vi "motor_stepping_diag_correct.vi"(0 "Initial Voltage (V)":dbl, 1 "Voltage Step (V)":dbl, 2 "First?":bool, 3 "Steps":dbl, 5 "Final Voltage (V)":dbl, 7 "Actual Voltage (V)  in":dbl, 9 "Final Voltage (V) 2":dbl, 11 "error in (no error)":errorcluster, 12 "Voltage Step2":dbl, 14 "Physical Channel":tag="Dev1/ao0") -> (4 "Actual Voltage (V)":dbl, 6 "Boolean":bool, 15 "error out":errorcluster)   [LabVIEW 2015]
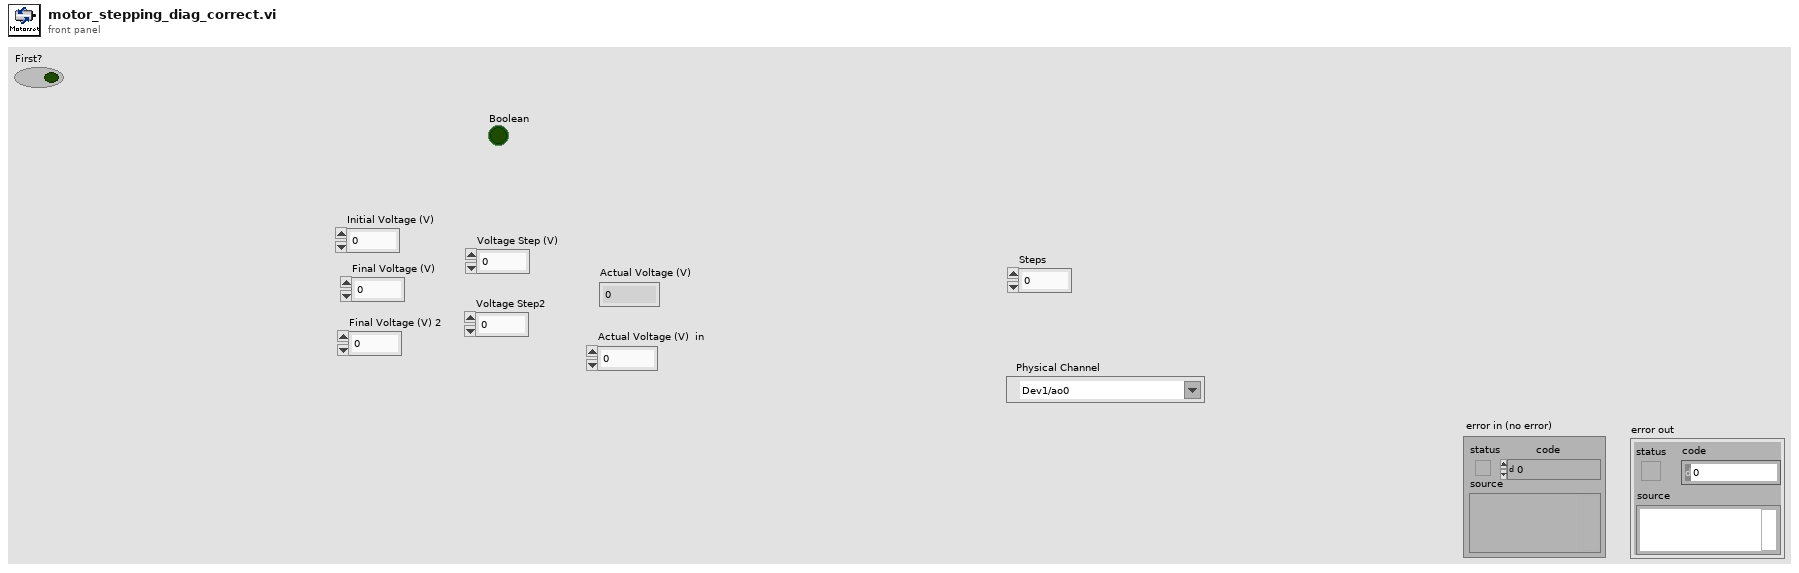
[diagram p1: front panel]
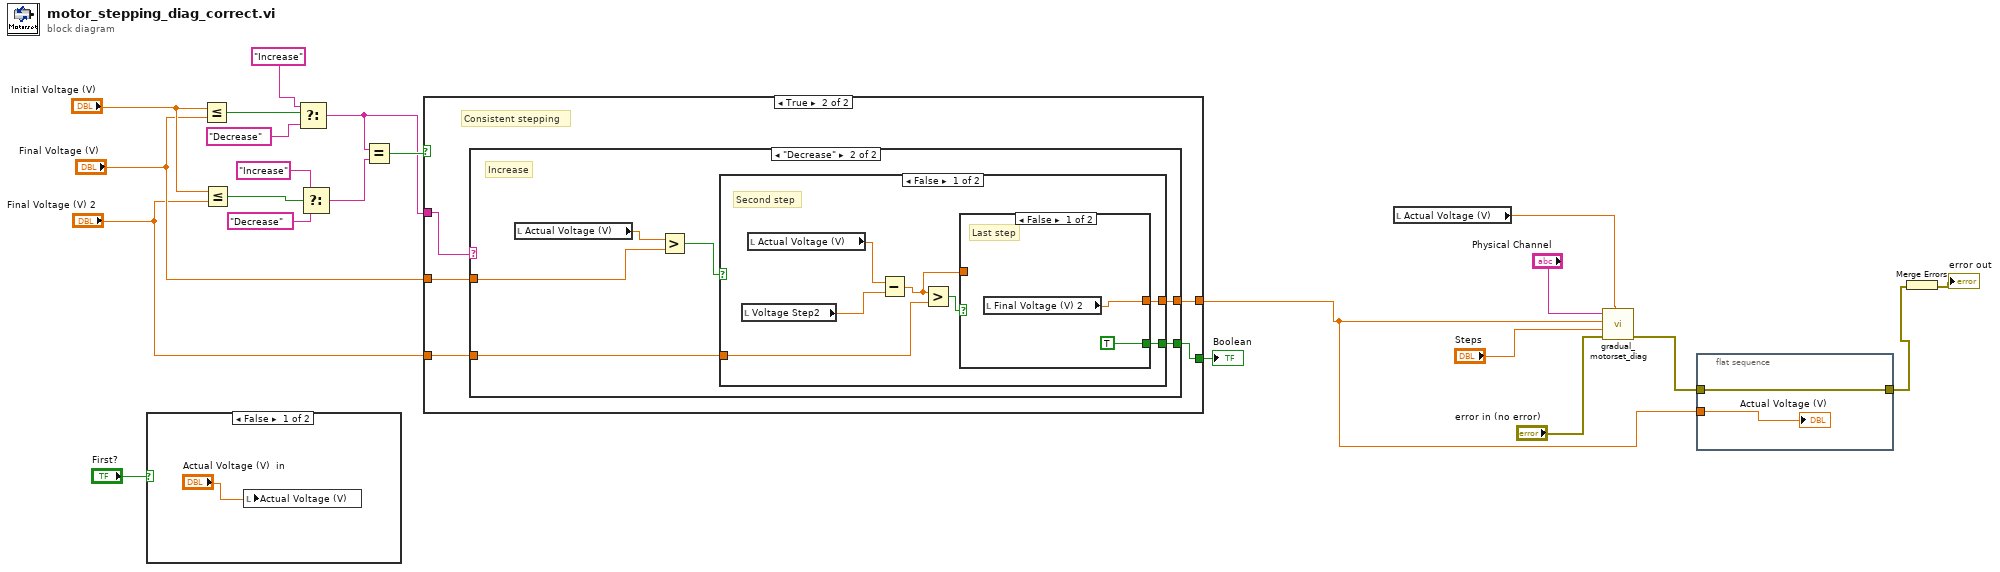
[diagram p0: block diagram]
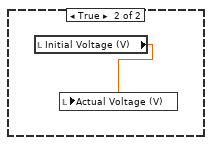
[diagram p2: hidden frame]
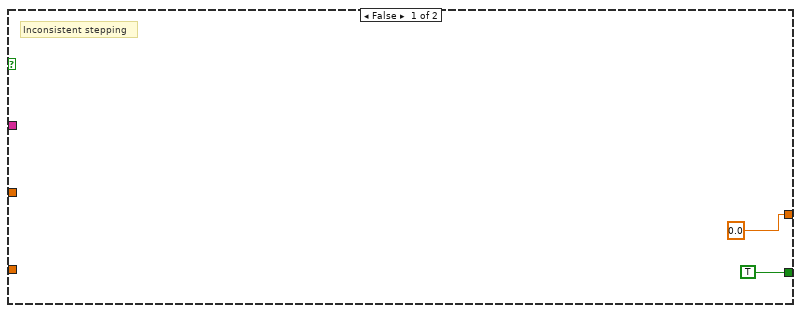
[diagram p3: hidden frame]
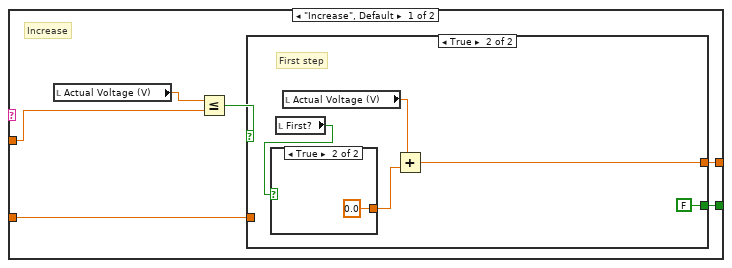
[diagram p4: hidden frame]
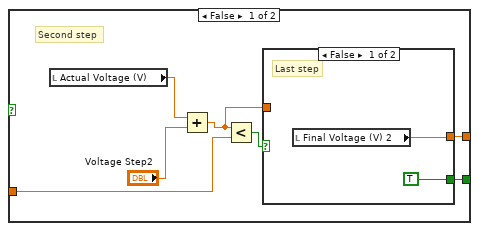
[diagram p5: hidden frame]
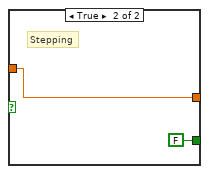
[diagram p6: hidden frame]
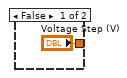
[diagram p7: hidden frame]
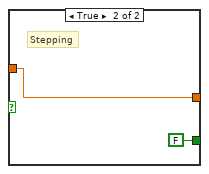
[diagram p8: hidden frame]
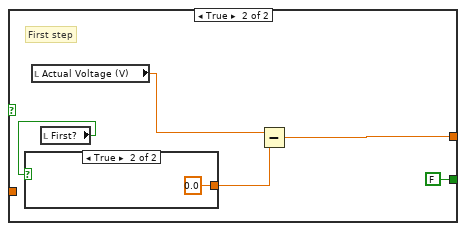
[diagram p9: hidden frame]
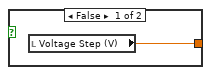
[diagram p10: hidden frame]
diagram:
  n1 = case shown="False" "First?" {
    frame False {
      n2 = local write "Actual Voltage (V)"("Actual Voltage (V)  in") -> ()
    }
    frame True {
      n3 = local read "Initial Voltage (V)"() -> (w24:dbl)
      n4 = local write "Actual Voltage (V)"(w24) -> ()
    }
  }
  n5 = Less Or Equal?(x="Initial Voltage (V)", y="Final Voltage (V)") -> (x <= y?=w20:bool)
  n6 = Less Or Equal?(x="Initial Voltage (V)", y="Final Voltage (V) 2") -> (x <= y?=w19:bool)
  n7 = Select(t="Increase", s=w20, f="Decrease") -> (s? t:f=w14:string)
  n8 = Select(t="Increase", s=w19, f="Decrease") -> (s? t:f=w13:string)
  n9 = Equal?(x=w14, y=w13) -> (x = y?=w15:bool)
  n10 = case shown="True" w15 {
    tunnel: w14 -> [_ w31]
    tunnel: "Final Voltage (V)" -> [_ w30]
    tunnel: [0.0 ("Actual Voltage (V)") w29] -> w4
    tunnel: "Final Voltage (V) 2" -> [_ w28]
    tunnel: [TRUE w27] -> w10
    frame False {
      # "Inconsistent stepping"
    }
    frame True {
      # "Consistent stepping"
      n11 = case shown="\"Decrease\"" w31 {
        tunnel: w30 -> [w35 w56]
        tunnel: [w34 w59] -> w29
        tunnel: w28 -> [w33 w58]
        tunnel: [w32 w57] -> w27
        frame "Increase", Default {
          # "Increase"
          n12 = local read "Actual Voltage (V)"() -> (w37:dbl)
          n13 = Less Or Equal?(x=w37, y=w35) -> (x <= y?=w36:bool)
          n14 = case shown="True" w36 {
            tunnel: [w40 w51] -> w34
            tunnel: w33 -> [w43 _]
            tunnel: [w38 FALSE] -> w32
            frame False {
              # "Second step"
              n15 = local read "Actual Voltage (V)"() -> (w39:dbl)
              n16 = Add(x=w39, y="Voltage Step2") -> (x+y=w41:dbl)
              n17 = Less?(x=w41, y=w43) -> (x < y?=w42:bool)
              n18 = case shown="False" w42 {
                tunnel: w41 -> [_ w48]
                tunnel: [w45 w48] -> w40
                tunnel: [TRUE FALSE] -> w38
                frame False {
                  # "Last step"
                  n19 = local read "Final Voltage (V) 2"() -> (w45:dbl)
                }
                frame True {
                  # "Stepping"
                }
              }
            }
            frame True {
              # "First step"
              n20 = local read "First?"() -> (w49:bool)
              n21 = case shown="True" w49 {
                tunnel: ["Voltage Step (V)" 0.0 ("Voltage Step (V)")] -> w53
                frame False {
                }
                frame True {
                }
              }
              n22 = local read "Actual Voltage (V)"() -> (w52:dbl)
              n23 = Add(x=w52, y=w53) -> (x+y=w51:dbl)
            }
          }
        }
        frame "Decrease" {
          # "Increase"
          n24 = local read "Actual Voltage (V)"() -> (w61:dbl)
          n25 = Greater?(x=w61, y=w56) -> (0:w60:bool)
          n26 = case shown="False" w60 {
            tunnel: [w65 w76] -> w59
            tunnel: w58 -> [w68 _]
            tunnel: [w63 FALSE] -> w57
            frame False {
              # "Second step"
              n27 = local read "Voltage Step2"() -> (w62:dbl)
              n28 = local read "Actual Voltage (V)"() -> (w64:dbl)
              n29 = Subtract(x=w64, y=w62) -> (x-y=w66:dbl)
              n30 = Greater?(x=w66, y=w68) -> (0:w67:bool)
              n31 = case shown="False" w67 {
                tunnel: w66 -> [_ w72]
                tunnel: [w69 w72] -> w65
                tunnel: [TRUE FALSE] -> w63
                frame False {
                  # "Last step"
                  n32 = local read "Final Voltage (V) 2"() -> (w69:dbl)
                }
                frame True {
                  # "Stepping"
                }
              }
            }
            frame True {
              # "First step"
              n33 = local read "Actual Voltage (V)"() -> (w77:dbl)
              n34 = local read "First?"() -> (w73:bool)
              n35 = case shown="True" w73 {
                tunnel: [w78 0.0 ("Voltage Step (V)")] -> w74
                frame False {
                  n36 = local read "Voltage Step (V)"() -> (w78:dbl)
                }
                frame True {
                }
              }
              n37 = Subtract(x=w77, y=w74) -> (x-y=w76:dbl)
            }
          }
        }
      }
    }
  }
  "Boolean" <- w10
  n38 = local read "Actual Voltage (V)"() -> (w5:dbl)
  n39 = call "gradual_motorset_diag.vi"("Initial Voltage (V)"=w5, "error in (no error)"="error in (no error)", "Steps"="Steps", "Next Voltage (V)"=w4, "Physical Channel"="Physical Channel") -> ("error out"=w2:errorcluster)  [unwired: 6 in]
  n40 = flat-sequence {
    tunnel: w4 -> [w81]
    tunnel: w2 -> [w80]
    tunnel: [w80] -> w1
    frame #0 {
      "Actual Voltage (V)" <- w81
    }
  }
  n41 = Merge Errors(w1) -> (→"error out":errorcluster)
